vi "Sensor_Conf_RW.vi"(7 "Mode":enum16{"Read", "Write"}(ring), 8 "error in":errorcluster, 10 "Section":string="system", 11 "Sensor_IN":T1) -> (0 "error out":errorcluster, 3 "Sensor_OUT":T1)   [LabVIEW 2020]
uses:
  Sensor.ctl
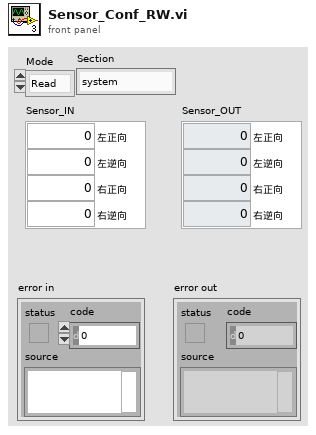
[diagram p1: front panel]
types:
  T1 = typedef "Sensor.ctl" = cluster{"左正向":dbl, "左逆向":dbl, "右正向":dbl, "右逆向":dbl}
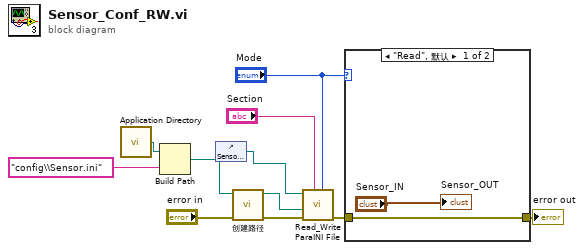
[diagram p0: block diagram]
diagram:
  n1 = call <vilib>:"Application Directory.vi"() -> ("Application Directory"=w11:path)
  n2 = Build Path(base path=w11, name or relative path="config\\Sensor.ini" ("名称或相对路径")) -> (appended path=w5:path)
  n3 = control-ref of="Sensor_IN"() -> (w1:refnum<vi>)
  n4 = call "创建路径.vi"("error in (no error)"="error in", "path"=w5) -> ("error out"=w2:errorcluster, "path out"=w4:path)  [unwired: 8 in]
  n5 = call "Read_Write ParaINI File.vi"("Mode"="Mode", "Section"="Section", "error in"=w2, "Filepath"=w4, "Ctl Refnum"=w1) -> ("error out"=w7:errorcluster)  [unwired: 6 in]
  n6 = case shown="\"Read\", 默认" "Mode" {
    tunnel: w7 -> [w13 w14]
    tunnel: [w13 w14] -> w6
    frame "Read", Default {
      "Sensor_OUT" <- "Sensor_IN"
    }
    frame "Write" {
    }
  }
  "error out" <- w6
